vi "SimPID.vi"(7 "Range":dbl, 8 "Position":dbl, 9 "Set Point":dbl, 10 "Gain":dbl) -> (0 "On Target":bool, 3 "result":dbl)   [LabVIEW 2011]
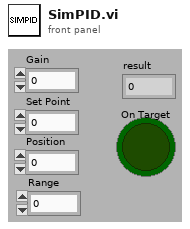
[diagram p1: front panel]
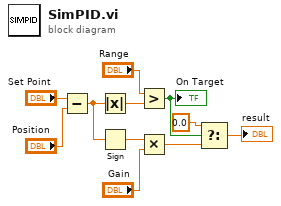
[diagram p0: block diagram]
diagram:
  n1 = Subtract(x="Set Point", y="Position") -> (x-y=w8:dbl)
  n2 = Absolute Value(x=w8) -> (abs(x)=w11:dbl)
  n3 = Sign(1:w8) -> (0:w7:dbl)
  n4 = Greater?(x="Range", y=w11) -> (0:w10:bool)
  "On Target" <- w10
  n5 = Multiply(x=w7, y="Gain") -> (x*y=w6:dbl)
  n6 = Select(t=0.0, s=w10, f=w6) -> (s? t:f=→"result":dbl)
